vi "Lang Set Main Page.vi"(8 "error in (no error)":errorcluster, 10 "Main":T1, 11 "Configuration Window in":refnum<class "Configuration Window.lvclass">) -> (0 "error out":errorcluster, 3 "Configuration Window out":refnum<class "Configuration Window.lvclass">)   [LabVIEW 2018, in "Configuration Window.lvlib" / "Configuration Window.lvclass"]
uses:
  Configuration Window.lvclass
  Framework/Framework/Const Lang CfgWnd Main.ctl
  Framework/Framework/Const Lang Property.ctl
  Configuration Window.lvclass/Configuration Window.ctl
  Framework/Framework/Framework.lvclass
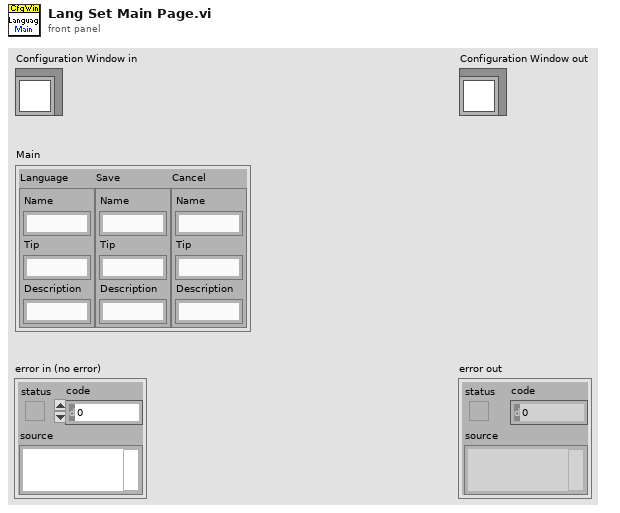
[diagram p1: front panel]
types:
  T1 = typedef "Framework.lvlib/Framework.lvclass/Const Lang CfgWnd Main.ctl" = cluster{"Language":T2, "Save":T2, "Cancel":T2}
  T2 = typedef "Framework.lvlib/Framework.lvclass/Const Lang Property.ctl" = cluster{"Name":string, "Tip":string, "Description":string}
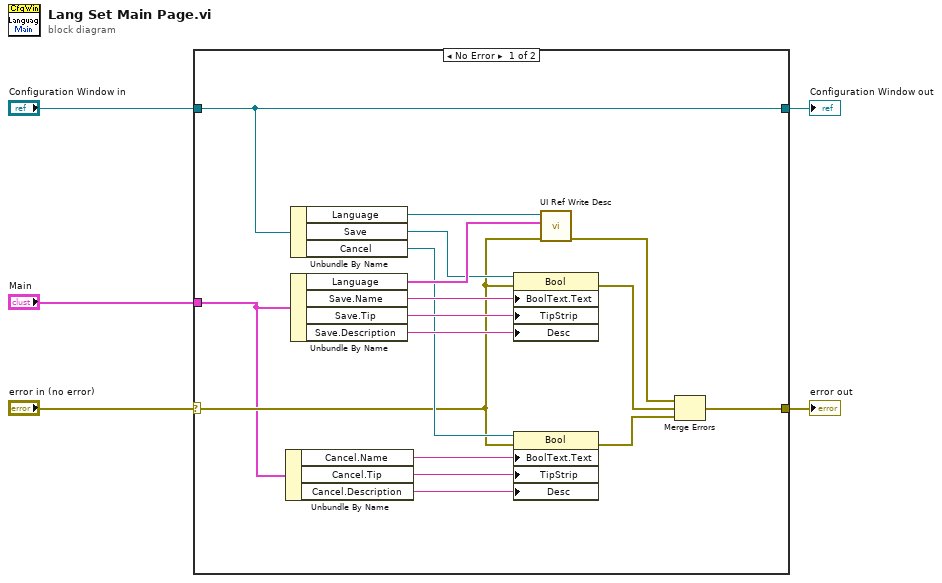
[diagram p0: block diagram]
diagram:
  n1 = case shown="No Error" "error in (no error)" {
    selector: "error in (no error)" -> [w12 w24]
    tunnel: [w20 w24] -> w4
    tunnel: [w22 w23] -> w2
    tunnel: "Configuration Window in" -> [w22 w23]
    tunnel: "Main" -> [w11 _]
    frame No Error {
      n2 = Unbundle By Name(w11) -> ("Cancel.Name"=w10:string, "Cancel.Tip"=w9:string, "Cancel.Description"=w8:string)
      n3 = Unbundle By Name(w22) -> ("Language"=w19:refnum<vi>, "Save"=w17:refnum<vi>, "Cancel"=w13:refnum<vi>)
      n4 = Unbundle By Name(w11) -> ("Language"=w18:T2, "Save.Name"=w16:string, "Save.Tip"=w15:string, "Save.Description"=w14:string)
      n5 = property class="Bool"(reference=w17, error in=w12, "BoolText.Text"=w16, "TipStrip"=w15, "Desc"=w14) -> (error out=w7:errorcluster)  [unwired: 1 out]
      n6 = property class="Bool"(reference=w13, error in=w12, "BoolText.Text"=w10, "TipStrip"=w9, "Desc"=w8) -> (error out=w6:errorcluster)  [unwired: 1 out]
      n7 = call "UI Ref Write Desc.vi"("error in (no error)"=w12, "UI Property"=w18, "UI Ref"=w19) -> ("error out"=w21:errorcluster)  [unwired: 8 in]
      n8 = Merge Errors(w21, w7, w6) -> (w20:errorcluster)
    }
    frame Error {
    }
  }
  "error out" <- w4
  "Configuration Window out" <- w2
